vi "PH_Beckhoff_PP_Control.PC Set PSDB Data.vi"(0 "VI in":refnum<vi>, 2 "PHELIX Subsystem":T1 items=["Miscellaneous", "fs-Frontend", "ns-Frontend", "PreAmp", "MainAmp", "MAS", "COS", "Beamline", "Experiment Laserbay", "Experiment Laserlabor", "Experiment Z6", "Timing", "Pulsed Power"], 5 "error in (no error)":errorcluster) -> (14 "VI out":refnum<vi>, 19 "error out":errorcluster)   [LabVIEW 2014, in "PH_Beckhoff_PP_Control.lvlib"]
uses:
  PH_Beckhoff_PP_Control.lvlib
  PH_Basics/PH_PSDBWriter/PH_PSDBWriter.PHELIX-Subsystems.ctl
  PH_Basics/PH_PSDBWriter/PH_PSDBWriter.Thread Commands.ctl
  PH_Basics/PH_PSDBWriter/PH_PSDBWriter.lvlib
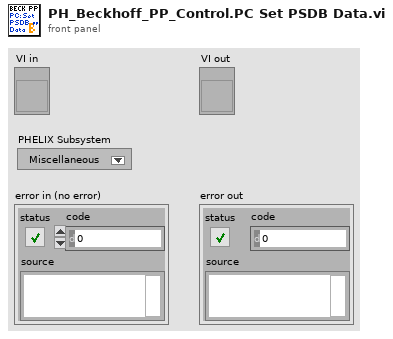
[diagram p1: front panel]
types:
  T1 = typedef "PH_PSDBWriter.lvlib/PH_PSDBWriter.PHELIX-Subsystems.ctl" = i32
  T2 = typedef "PH_Beckhoff_PP_Control.lvlib/PH_Beckhoff_PP_Control.i attribute.ctl" = cluster{"PP Conductivity Control":cluster{"PSDB":cluster{"Status Service ID":i32, "Instance ID":i32, "Data Status":T3, "Ref Status":refnum<vi>, "Error Code":i32}, "Status":cluster{"GUI Ref":refnum<vi>, "Status Service ID":i32, "Status":T4}, "DIs":cluster{"Device on":cluster{"GUI Ref":refnum<vi>, "# in Data":i32}, "Conductivity ok":cluster{"GUI Ref":refnum<vi>, "# in Data":i32}, "Temperature ok":cluster{"GUI Ref":refnum<vi>, "# in Data":i32}, "Alarm":cluster{"GUI Ref":refnum<vi>, "# in Data":i32}}, "PSDB Thread":cluster{"Ref":refnum<vi>, "Q-Ref":refnum<queue>}}, "PP Mercury Control":cluster{"PSDB":cluster{"Status Service ID":i32, "Instance ID":i32, "Data Status":T3, "Ref Status":refnum<vi>, "Error Code":i32}, "Status":cluster{"GUI Ref":refnum<vi>, "Status Service ID":i32, "Status":T4}, "on since:":cluster{"GUI Ref":refnum<vi>, "Service ID":i32, "Time":string}, "DIs":cluster{"Device on":cluster{"GUI Ref":refnum<vi>, "# in Data":i32}, "Alarm":cluster{"GUI Ref":refnum<vi>, "# in Data":i32}}, "AIs":cluster{"Concentration":cluster{"GUI Ref":refnum<vi>, "# in Data":i32}}, "PSDB Thread":cluster{"Ref":refnum<vi>, "Q-Ref":refnum<queue>}}, "PSDB":cluster{"Shot #":i32, "Subsystem":T1}, "PSDB Credentials":T5}
  T3 = typedef "PH_PSDBWriter.lvlib/PH_PSDBWriter.Data Status.ctl" = i16
  T4 = typedef "PH_StatusHandler.lvlib/PH_StatusHandler.Status.ctl" = i16
  T5 = typedef "PH_Common.lvlib/PH_Connection.PSDB Credentials.ctl" = cluster{"PW":string, "ID":string, "DS":string}
  T6 = typedef "PH_PSDBWriter.lvlib/PH_PSDBWriter.Thread Commands.ctl" = u16
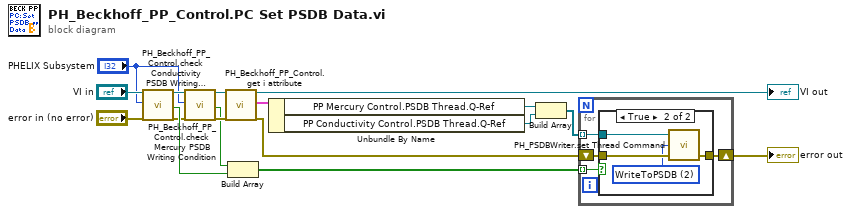
[diagram p0: block diagram]
diagram:
  n1 = call "PH_Beckhoff_PP_Control.check Conductivity PSDB Writing Condition.vi"("i ref in"="VI in", "wanted Subsystem"="PHELIX Subsystem", "error IO"="error in (no error)") -> ("i ref out"=w2:refnum<vi>, "write Conductivity Data to PSDB?"=w5:bool, "error out"=w3:errorcluster)  [unwired: 14 in]
  n2 = call "PH_Beckhoff_PP_Control.check Mercury PSDB Writing Condition.vi"("i ref in"=w2, "wanted Subsystem"="PHELIX Subsystem", "error IO"=w3) -> ("i ref out"=w10:refnum<vi>, "write Mercury Data to PSDB?"=w4:bool, "error out"=w12:errorcluster)  [unwired: 14 in]
  n3 = call "PH_Beckhoff_PP_Control.get i attribute.vi"("i ref in"=w10, "error in (no error)"=w12) -> ("i ref out"=→"VI out":refnum<vi>, "i attribute"=w14:T2, "error out"=w13:errorcluster)  [unwired: 15 in]
  n4 = Build Array(w4, w5) -> (w6:bool[])
  n5 = Unbundle By Name(w14) -> ("PP Mercury Control.PSDB Thread.Q-Ref"=w15:refnum<queue>, "PP Conductivity Control.PSDB Thread.Q-Ref"=w16:refnum<queue>)
  n6 = Build Array(w15, w16) -> (w17:refnum<queue>[])
  n7 = for {
    tunnel: w6 -> [w21] mode=indexing
    shift-right: [w19] -> w7
    shift-left: w13 -> [w20]
    tunnel: w17 -> [w18] mode=indexing
    n8 = case shown="True" w21 {
      tunnel: w20 -> [w22 w26]
      tunnel: [w22 w25] -> w19
      tunnel: w18 -> [_ w23]
      frame False {
      }
      frame True {
        w24 = T6 2 items=["None", "GetInstanceID", "WriteToPSDB"] ("PSDB Thread Command")
        n9 = call "PH_PSDBWriter.set Thread Command.vi"("error in (no error)"=w26, "PSDB Thread Command"=w24, "Queue in"=w23) -> ("error out"=w25:errorcluster)  [unwired: 2 in]
      }
    }
  }
  "error out" <- w7
